vi "sub2.vi"(11 "String in":string) -> (3 "String out":string)   [LabVIEW 2018]
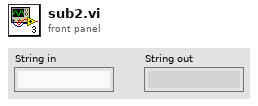
[diagram p1: front panel]
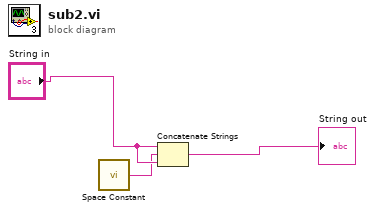
[diagram p0: block diagram]
diagram:
  n1 = call <vilib>:"Space Constant.vi"() -> ("String"=w1:string)
  n2 = Concatenate Strings("String in", w1, "String in") -> (→"String out":string)
